vi "Three part faster sub.vi"() -> ()   [LabVIEW 2009]
uses:
  <vilib>/vision/Image Controls.llb/IMAQ Image.ctl
  <vilib>/Instr/_visa.llb/VISA Configure Serial Port (Instr).vi
  <vilib>/vision/NI_Vision_Development_Module.lvlib
panel:
  out "Image 2":T1(plugin-control)
  in  "Orange Bass":T2={"Global Rectangle"=[220, 302, 227, 392], "Contours"=[{"ID"=enum."External", "Type"=2, "Coordinates"=[226, 391, 220, 302]}]} {"Contours"."Type" items=["No Selection", "Point", "Line", "Rectangle", "Oval", "Polygon", "Freehand Region", "Annulus", "Unused2", "Unused3", "Broken Line", "Freehand Line", "Rotated Rectangle"]}
  in  "Blue Bass":T2={"Global Rectangle"=[192, 292, 199, 386], "Contours"=[{"ID"=enum."External", "Type"=2, "Coordinates"=[192, 385, 198, 292]}]} {"Contours"."Type" items=["No Selection", "Point", "Line", "Rectangle", "Oval", "Polygon", "Freehand Region", "Annulus", "Unused2", "Unused3", "Broken Line", "Freehand Line", "Rotated Rectangle"]}
  in  "playtime":dbl=30.0
  out "decimal integer string 2":string
  out "number 2":u32
  out "cluster 2":T3
  in  "Orange Guitar":T2={"Global Rectangle"=[587, 282, 628, 378], "Contours"=[{"ID"=enum."External", "Type"=2, "Coordinates"=[627, 377, 587, 282]}]} {"Contours"."Type" items=["No Selection", "Point", "Line", "Rectangle", "Oval", "Polygon", "Freehand Region", "Annulus", "Unused2", "Unused3", "Broken Line", "Freehand Line", "Rotated Rectangle"]}
  in  "Yellow Guitar":T2={"Global Rectangle"=[546, 282, 563, 376], "Contours"=[{"ID"=enum."External", "Type"=2, "Coordinates"=[562, 375, 546, 282]}]} {"Contours"."Type" items=["No Selection", "Point", "Line", "Rectangle", "Oval", "Polygon", "Freehand Region", "Annulus", "Unused2", "Unused3", "Broken Line", "Freehand Line", "Rotated Rectangle"]}
  in  "Green Guitar":T2={"Global Rectangle"=[498, 284, 505, 376], "Contours"=[{"ID"=enum."External", "Type"=2, "Coordinates"=[498, 375, 504, 284]}]} {"Contours"."Type" items=["No Selection", "Point", "Line", "Rectangle", "Oval", "Polygon", "Freehand Region", "Annulus", "Unused2", "Unused3", "Broken Line", "Freehand Line", "Rotated Rectangle"]}
  in  "Blue Guitar":T2={"Global Rectangle"=[569, 290, 594, 372], "Contours"=[{"ID"=enum."External", "Type"=2, "Coordinates"=[593, 371, 569, 290]}]} {"Contours"."Type" items=["No Selection", "Point", "Line", "Rectangle", "Oval", "Polygon", "Freehand Region", "Annulus", "Unused2", "Unused3", "Broken Line", "Freehand Line", "Rotated Rectangle"]}
  in  "Red Guitar":T2={"Global Rectangle"=[526, 284, 530, 370], "Contours"=[{"ID"=enum."External", "Type"=2, "Coordinates"=[529, 369, 526, 284]}]} {"Contours"."Type" items=["No Selection", "Point", "Line", "Rectangle", "Oval", "Polygon", "Freehand Region", "Annulus", "Unused2", "Unused3", "Broken Line", "Freehand Line", "Rotated Rectangle"]}
  out "Yellow Guitar LED":bool
  out "Green Guitar LED":bool
  out "Red Guitar LED":bool
  out "Blue Guitar LED":bool
  out "Orange Guitar LED":bool
  out "Orange Bass LED":bool
  in  "Green Bass":T2={"Global Rectangle"=[100, 292, 131, 371], "Contours"=[{"ID"=enum."External", "Type"=2, "Coordinates"=[100, 370, 130, 292]}]} {"Contours"."Type" items=["No Selection", "Point", "Line", "Rectangle", "Oval", "Polygon", "Freehand Region", "Annulus", "Unused2", "Unused3", "Broken Line", "Freehand Line", "Rotated Rectangle"]}
  in  "Red Bass":T2={"Global Rectangle"=[129, 294, 154, 376], "Contours"=[{"ID"=enum."External", "Type"=2, "Coordinates"=[129, 375, 153, 294]}]} {"Contours"."Type" items=["No Selection", "Point", "Line", "Rectangle", "Oval", "Polygon", "Freehand Region", "Annulus", "Unused2", "Unused3", "Broken Line", "Freehand Line", "Rotated Rectangle"]}
  in  "Yellow Bass":T2={"Global Rectangle"=[160, 295, 175, 378], "Contours"=[{"ID"=enum."External", "Type"=2, "Coordinates"=[160, 377, 174, 295]}]} {"Contours"."Type" items=["No Selection", "Point", "Line", "Rectangle", "Oval", "Polygon", "Freehand Region", "Annulus", "Unused2", "Unused3", "Broken Line", "Freehand Line", "Rotated Rectangle"]}
  out "Yellow Bass LED":bool
  out "Green Bass LED":bool
  out "Red Bass LED":bool
  out "Blue Bass LED":bool
  in  "Mask":T2 {"Contours"."Type" items=["No Selection", "Point", "Line", "Rectangle", "Oval", "Polygon", "Freehand Region", "Annulus", "Unused2", "Unused3", "Broken Line", "Freehand Line", "Rotated Rectangle"]}
  in  "Red Line":T2={"Global Rectangle"=[300, 297, 320, 380], "Contours"=[{"ID"=enum."External", "Type"=2, "Coordinates"=[300, 379, 319, 297]}]} {"Contours"."Type" items=["No Selection", "Point", "Line", "Rectangle", "Oval", "Polygon", "Freehand Region", "Annulus", "Unused2", "Unused3", "Broken Line", "Freehand Line", "Rotated Rectangle"]}
  out "Red Drum":bool
  in  "Blue Line":T2={"Global Rectangle"=[374, 278, 383, 377], "Contours"=[{"ID"=enum."External", "Type"=2, "Coordinates"=[382, 376, 374, 278]}]} {"Contours"."Type" items=["No Selection", "Point", "Line", "Rectangle", "Oval", "Polygon", "Freehand Region", "Annulus", "Unused2", "Unused3", "Broken Line", "Freehand Line", "Rotated Rectangle"]}
  in  "Green Line":T2={"Global Rectangle"=[406, 309, 423, 383], "Contours"=[{"ID"=enum."External", "Type"=2, "Coordinates"=[422, 382, 406, 309]}]} {"Contours"."Type" items=["No Selection", "Point", "Line", "Rectangle", "Oval", "Polygon", "Freehand Region", "Annulus", "Unused2", "Unused3", "Broken Line", "Freehand Line", "Rotated Rectangle"]}
  out "Green Drum":bool
  in  "Yellow Line":T2={"Global Rectangle"=[342, 292, 349, 377], "Contours"=[{"ID"=enum."External", "Type"=2, "Coordinates"=[342, 376, 348, 292]}]} {"Contours"."Type" items=["No Selection", "Point", "Line", "Rectangle", "Oval", "Polygon", "Freehand Region", "Annulus", "Unused2", "Unused3", "Broken Line", "Freehand Line", "Rotated Rectangle"]}
  out "cluster":T3
  in  "VISA resource name":refnum<visa-resource-name>
  out "number":u32
  out "decimal integer string":string
  out "Image Dst Out":T1
  out "Yellow Drum":bool
  out "Frame Number":i32
  in  "Frame Start":i32
  out "Blue Drum":bool
  in  "stop":bool
  in  "AVI Path":path
  # "Drums"
  # "Bass"
  # "Guitar"
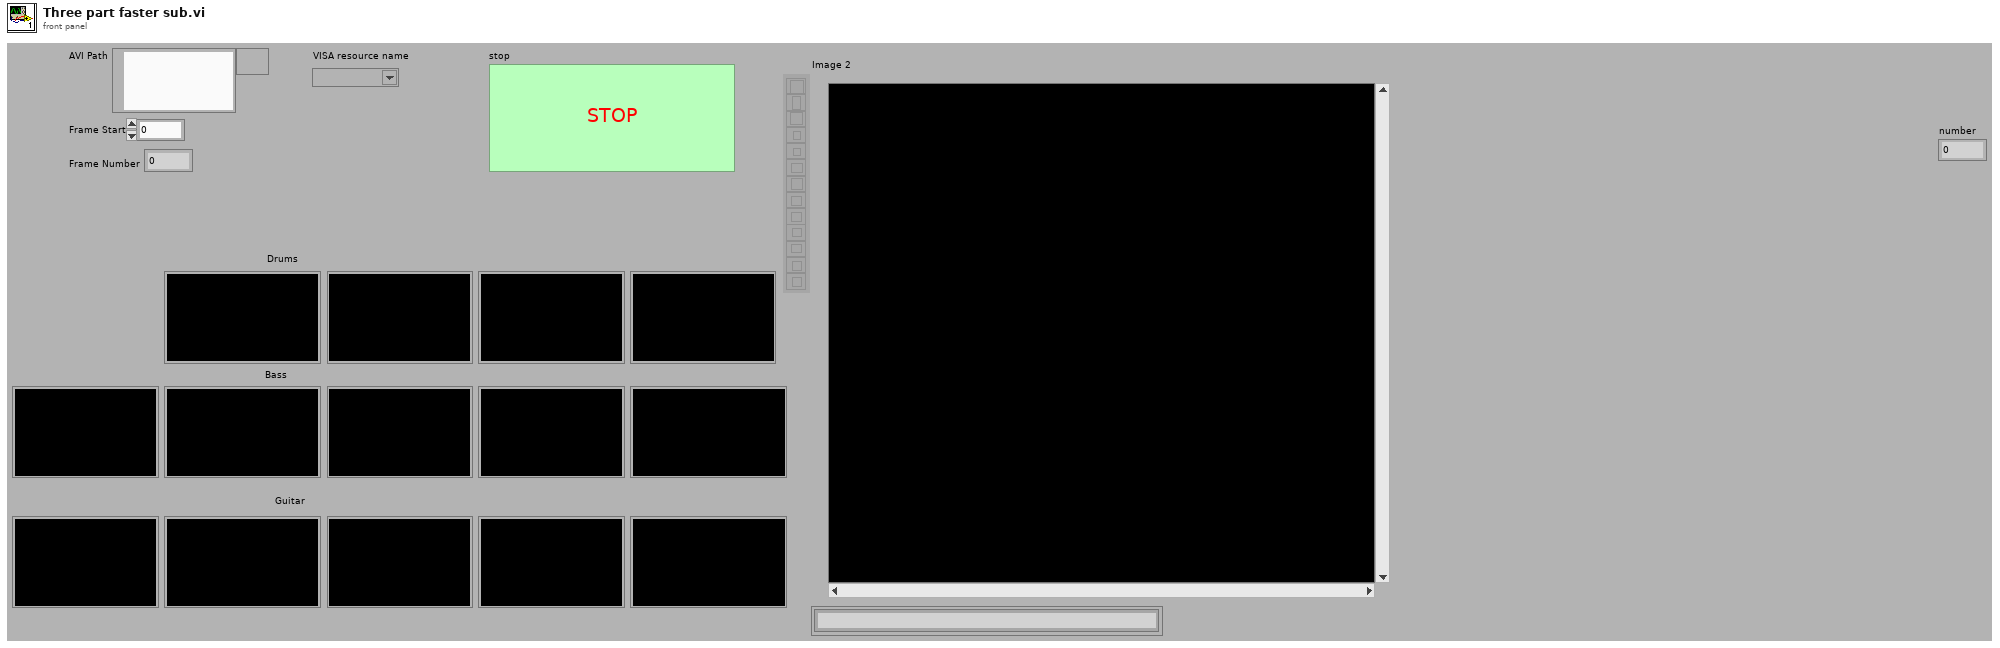
[diagram p1: front panel]
types:
  T1 = typedef "IMAQ Image.ctl" = refnum<image>
  T2 = cluster{"Global Rectangle":i32[], "Contours":cluster{"ID":enum32{"External", "Internal"}, "Type":u32, "Coordinates":i32[]}[]}
  T3 = cluster{"[0]":bool, "[1]":bool, "[2]":bool, "[3]":bool, "[4]":bool, "[5]":bool, "[6]":bool, "[7]":bool, "[8]":bool}
  T4 = typedef "Image Type" = u32
  T5 = typedef "AviRefnum.ctl" = refnum<k1>
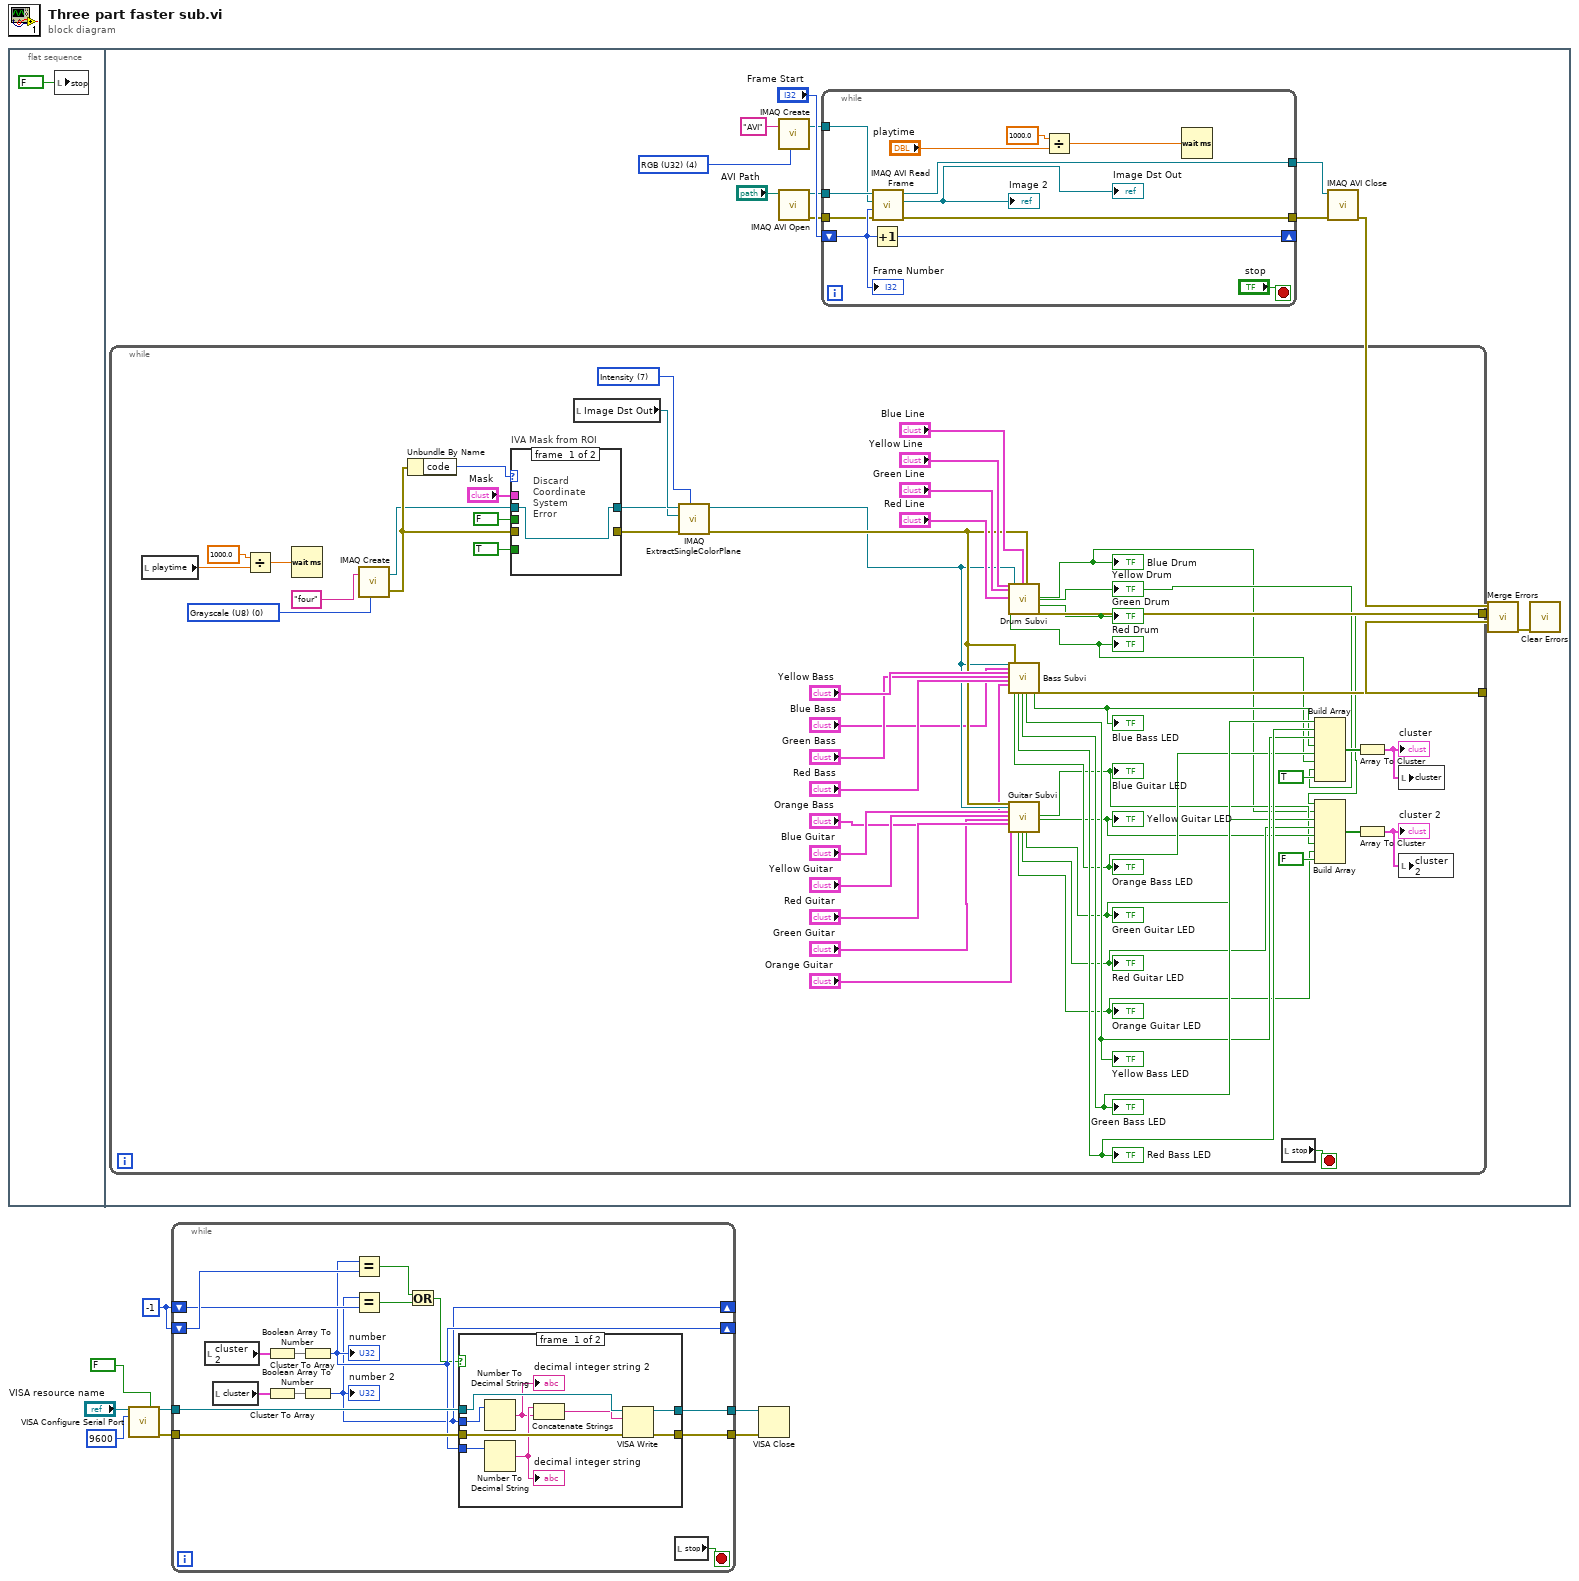
[diagram p0: block diagram]
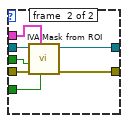
[diagram p3: hidden frame]
diagram:
  w1 = -1
  n1 = flat-sequence {
    frame #0 {
      n2 = local write "stop"(FALSE ("stop")) -> ()
    }
    frame #1 {
      w14 = T4 4 items=["Grayscale (U8)", "Grayscale (I16)", "Grayscale (SGL)", "Complex (CSG)", "RGB (U32)", "HSL (U32)", "RGB (U64)", "Grayscale (U16)"] ("Image Type")
      n3 = while {
        tunnel: [w61] -> w11
        tunnel: [w51] -> w10
        stop <- w75 stop-if-true
        w71 = T4 0 items=["Grayscale (U8)", "Grayscale (I16)", "Grayscale (SGL)", "Complex (CSG)", "RGB (U32)", "HSL (U32)", "RGB (U64)", "Grayscale (U16)"] ("Image Type")
        w76 = 7 items=["Red", "Green", "Blue", "Hue", "Saturation", "Luminance", "Value", "Intensity"] ("Color Plane")
        n4 = local read "playtime"() -> (w41:dbl)
        n5 = Divide(x=1000.0, y=w41) -> (x/y=w74:dbl)
        n6 = Wait (ms)(milliseconds to wait=w74) -> ()  [unwired: 1 out]
        n7 = call "IMAQ Create"("Image Name"="four", "Image Type"=w71) -> ("New Image"=w64:T1, "error out"=w65:errorcluster)  [unwired: 3 in]
        n8 = Unbundle By Name(w65) -> ("code"=w69:i32)
        n9 = case "IVA Mask from ROI" shown="Default" w69 {
          tunnel: "Mask" -> [_ w84]
          tunnel: TRUE ("Shrink") -> [_ w83]
          tunnel: w64 -> [w77 w82]
          tunnel: w65 -> [_ w81]
          tunnel: [_ w80] -> w66
          tunnel: [w77 w79] -> w62
          tunnel: FALSE ("Out / In") -> [_ w78]
          frame #0 {
            # "Discard\nCoordinate\nSystem\nError"
          }
          frame #1 {
            n10 = call <vilib>:"IVA Mask from ROI.vi"("Shrink"=w83, "ROI Descriptor"=w84, "error in (no error)"=w81, "Out / In"=w78, "Image Src"=w82) -> ("error out"=w80:errorcluster, "Image Out"=w79:T1)  [unwired: 5 out]
          }
        }
        n11 = local read "Image Dst Out"() -> (w72:T1)
        n12 = call "IMAQ ExtractSingleColorPlane"("Color Plane"=w76, "error in (no error)"=w66, "Image Dst"=w62, "Image Src"=w72) -> ("error out"=w50:errorcluster, "Image Dst Out"=w45:T1)  [unwired: 6 out]
        n13 = call "Drum Subvi.vi"("Yellow Line"="Yellow Line", "Green Line"="Green Line", "Red Line"="Red Line", "Image Dst Out"=w45, "Blue Line"="Blue Line", "error out"=w50) -> ("LED Red"=w26:bool, "Blue Drum 2"=w23:bool, "Yellow Drum"=w25:bool, "Green Drum"=w24:bool, "error out 2"=w61:errorcluster)  [unwired: 12 in, 5 out]
        "Yellow Drum" <- w25
        "Green Drum" <- w24
        "Red Drum" <- w26
        "Blue Drum" <- w23
        n14 = call "Bass Subvi.vi"("Image Dst Out"=w45, "Blue Bass 2"="Blue Bass", "Yellow Bass 2"="Yellow Bass", "Green Bass 2"="Green Bass", "Red Bass 2"="Red Bass", "Orange Bass 2"="Orange Bass", "error out"=w50) -> ("Orange Bass LED"=w32:bool, "Red Bass LED"=w35:bool, "Green Bass LED"=w36:bool, "Yellow Bass LED"=w34:bool, "Blue Bass LED"=w33:bool, "error out 2"=w51:errorcluster)  [unwired: 15 in]
        "Yellow Bass LED" <- w34
        "Green Bass LED" <- w36
        "Red Bass LED" <- w35
        "Blue Bass LED" <- w33
        "Orange Bass LED" <- w32
        n15 = call "Guitar Subvi.vi"("error out"=w50, "Image Dst Out"=w45, "Blue Guitar 2"="Blue Guitar", "Yellow Guitar 2"="Yellow Guitar", "Green Guitar 2"="Green Guitar", "Red Guitar 2"="Red Guitar", "Orange Guitar 2"="Orange Guitar") -> ("Orange Guitar LED"=w27:bool, "Red Guitar LED"=w30:bool, "Green Guitar LED"=w31:bool, "Blue Guitar LED"=w28:bool, "Yellow Guitar LED"=w29:bool)  [unwired: 16 in]
        "Yellow Guitar LED" <- w29
        "Green Guitar LED" <- w31
        "Red Guitar LED" <- w30
        "Blue Guitar LED" <- w28
        "Orange Guitar LED" <- w27
        n16 = local read "stop"() -> (w75:bool)
        n17 = Build Array(w36, w35, w34, w33, w32, w26, w25, TRUE ("element")) -> (w56:bool[])
        n18 = Build Array(w24, w23, w31, w30, w29, w28, w27, FALSE ("element")) -> (w43:bool[])
        n19 = Array To Cluster(array=w56) -> (cluster=w57:T3)
        "cluster" <- w57
        n20 = Array To Cluster(array=w43) -> (cluster=w42:T3)
        "cluster 2" <- w42
        n21 = local write "cluster"(w57) -> ()
        n22 = local write "cluster 2"(w42) -> ()
      }
      n23 = call "IMAQ Create"("Image Name"="AVI", "Image Type"=w14) -> ("New Image"=w12:T1)  [unwired: 3 in, 1 out]
      n24 = call "IMAQ AVI Open"("AVI Path"="AVI Path") -> ("error out"=w19:errorcluster, "Avi Refnum"=w20:T5)  [unwired: 9 in]
      n25 = while {
        tunnel: w20 -> [w96]
        tunnel: w19 -> [w88]
        tunnel: [w95] -> w21
        shift-right: [w90] -> _
        shift-left: "Frame Start" -> [w89]
        tunnel: [w87] -> w15
        tunnel: w12 -> [w86]
        stop <- "stop" stop-if-true
        n26 = Increment(x=w89) -> (x+1=w90:i32)
        n27 = call "IMAQ AVI Read Frame"("error in (no error)"=w88, "Frame Number"=w89, "Image"=w86, "Avi Refnum"=w96) -> ("error out"=w87:errorcluster, "Image Out"=→"Image Dst Out" →"Image 2":T1, "Avi Refnum (duplicate)"=w95:T5)  [unwired: 4 in, 1 out]
        n28 = Divide(x=1000.0, y="playtime") -> (x/y=w93:dbl)
        n29 = Wait (ms)(milliseconds to wait=w93) -> ()  [unwired: 1 out]
        "Frame Number" <- w89
      }
      n30 = call "IMAQ AVI Close"("error in (no error)"=w15, "Avi Refnum"=w21) -> ("error out"=w17:errorcluster)  [unwired: 9 in]
      n31 = call <vilib>:"Merge Errors.vi"("error in 3 (no error)"=w10, "error in 2 (no error)"=w11, "error in 1 (no error)"=w17) -> ("error out"=w16:errorcluster)  [unwired: 4 in]
      n32 = call <vilib>:"Clear Errors.vi"("error in (no error)"=w16) -> ()  [unwired: 6 in, 1 out]
    }
  }
  n33 = call-poly "VISA Configure Serial Port"("VISA resource name"="VISA resource name", "Enable Termination\nChar (T)"=FALSE ("Enable Termination\nChar (T)"), "baud rate (9600)"=u32 9600) -> ("VISA resource name out"=w8:refnum<visa-resource-name>, "error out"=w3:errorcluster)  [unwired: 11 in]
  n34 = while {
    shift-right: [w101] -> _
    shift-left: w1 -> [w112]
    tunnel: w8 -> [w111]
    tunnel: [w110] -> w7
    tunnel: w3 -> [w109]
    tunnel: [w108] -> w2
    shift-right: [w100] -> _
    shift-left: w1 -> [w104]
    stop <- w106 stop-if-true
    n35 = local read "cluster 2"() -> (w102:T3)
    n36 = local read "cluster"() -> (w103:T3)
    n37 = Cluster To Array(cluster=w102) -> (array=w107:bool[])
    n38 = Cluster To Array(cluster=w103) -> (array=w105:bool[])
    n39 = Boolean Array To Number(Boolean array=w107) -> (number=w101:u32)
    "number" <- w101
    n40 = Boolean Array To Number(Boolean array=w105) -> (number=w100:u32)
    "number 2" <- w100
    n41 = Equal?(x=w101, y=w112) -> (x = y?=w99:bool)
    n42 = Equal?(x=w100, y=w104) -> (x = y?=w98:bool)
    n43 = Or(x=w99, y=w98) -> (x .or. y?=w97:bool)
    n44 = case shown="False" w97 {
      tunnel: w111 -> [w121 w123]
      tunnel: [w120 w123] -> w110
      tunnel: w101 -> [w119 _]
      tunnel: w109 -> [w118 w122]
      tunnel: [w117 w122] -> w108
      tunnel: w100 -> [w116 _]
      frame #0 {
        n45 = Number To Decimal String(number=w116) -> (decimal integer string=w114:string)  [unwired: 1 in]
        "decimal integer string 2" <- w114
        n46 = Number To Decimal String(number=w119) -> (decimal integer string=w115:string)  [unwired: 1 in]
        "decimal integer string" <- w115
        n47 = Concatenate Strings(w115, w114) -> (w113:string)
        n48 = VISA Write(VISA resource name=w121, write buffer=w113, error in (no error)=w118) -> (VISA resource name out=w120:refnum<visa-resource-name>, error out=w117:errorcluster)  [unwired: 1 out]
      }
      frame #1 {
      }
    }
    n49 = local read "stop"() -> (w106:bool)
  }
  n50 = VISA Close(VISA resource name=w7, error in (no error)=w2) -> ()  [unwired: 1 out]
